vi "Initialise Web Client.vi"(8 "error in (no error)":errorcluster, 10 "Address":string) -> (0 "error out":errorcluster, 3 "Web Client out":refnum<class "Web Client.lvclass">)   [LabVIEW 2018, in "Collaborator.lvlib" / "Web Client.lvclass"]
uses:
  Web Client.lvclass
  Web Client.lvclass/Web Client.ctl
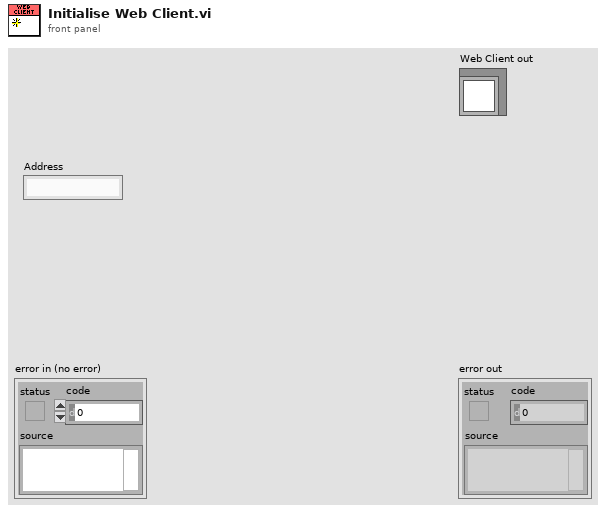
[diagram p1: front panel]
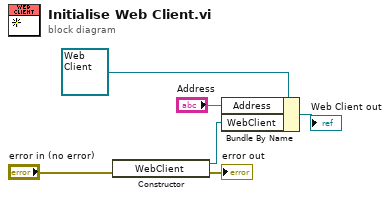
[diagram p0: block diagram]
diagram:
  n1 = constructor class="WebClient"(error in="error in (no error)") -> (reference out=w2:refnum<k24>, error out=→"error out":errorcluster)  [unwired: 2 in, 1 out]
  n2 = Bundle By Name(cluster=refnum<class "Web Client.lvclass"> refnum ("Web Client in"), "Address"="Address", "WebClient"=w2) -> (→"Web Client out":refnum<class "Web Client.lvclass">)
